vi "Create All Message Queues.vi"(8 "error in (no error)":errorcluster) -> (0 "error out":errorcluster, 3 "Message Queues out":T1)   [LabVIEW 2018, in "Message Queue.lvlib"]
doc: "This VI creates and initializes all the message queues for your application. If your application requires more than one message queue, right-click the \"Message Queues\" constant above and select Open Type Def. Add the new Message Queue(s) to the type definition, then initialize them in this VI."
uses:
  Message Queue.lvlib
  All Message Queues.ctl
  Message Cluster (enum).ctl
  Message (enum).ctl
  Message Cluster (string).ctl
  Enqueue Message (string).vi
  Enqueue Message (enum).vi
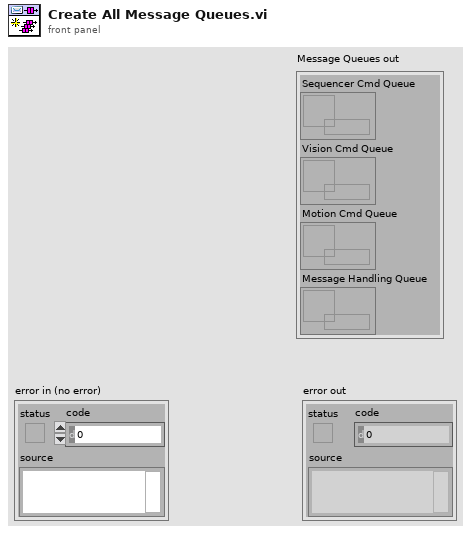
[diagram p1: front panel]
types:
  T1 = typedef "Message Queue.lvlib/All Message Queues.ctl" = cluster{"Sequencer Cmd Queue":refnum<queue>, "Vision Cmd Queue":refnum<queue>, "Motion Cmd Queue":refnum<queue>, "Message Handling Queue":refnum<queue>}
  T2 = typedef "Message Queue.lvlib/Message (enum).ctl" = enum16{"Initialize", "Idle", "Running", "Stop", "Pause", "Resume", "Load Sequence", "Exit"}
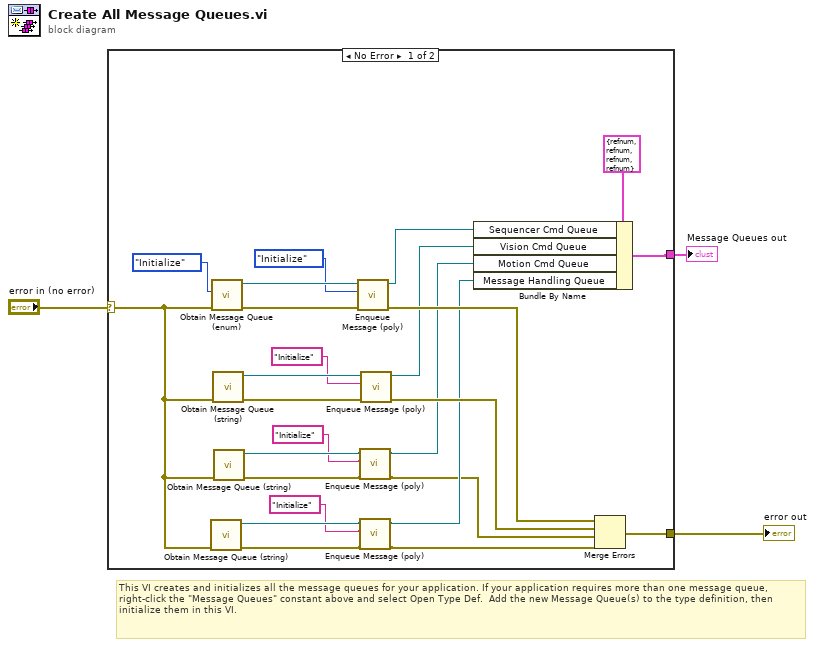
[diagram p0: block diagram]
diagram:
  # "This VI creates and initializes all the message queues for your application. If your application requires more than one message queue, right-click the \"Message Queues\" constant above and select Open Type Def.  Add the new Message Queue(s) to the type definition, then initialize them in this VI."
  n1 = case shown="No Error" "error in (no error)" {
    selector: "error in (no error)" -> [w5 w29]
    tunnel: [w26 w29] -> w3
    tunnel: [w27 _] -> w2
    frame No Error {
      n2 = call "Obtain Message Queue (string).vi"("error in (no error)"=w5) -> ("error out"=w13:errorcluster, "queue out"=w14:refnum<queue>)  [unwired: 9 in]
      n3 = call "Obtain Message Queue (enum).vi"("error in (no error)"=w5, "Message"=Message_(enum)."Initialize" ("Enum")) -> ("error out"=w25:errorcluster, "queue out"=w23:refnum<queue>)  [unwired: 8 in]
      n4 = call "Obtain Message Queue (string).vi"("error in (no error)"=w5) -> ("error out"=w20:errorcluster, "queue out"=w19:refnum<queue>)  [unwired: 9 in]
      n5 = call "Obtain Message Queue (string).vi"("error in (no error)"=w5) -> ("error out"=w9:errorcluster, "queue out"=w17:refnum<queue>)  [unwired: 9 in]
      n6 = call-poly "Enqueue Message (poly).vi"("error in (no error)"=w25, "Enum"=Message_(enum)."Initialize", "Message Queue"=w23) -> ("error out"=w24:errorcluster, "dup Message Queue"=w6:refnum<queue>)  [unwired: 7 in]
      n7 = call-poly "Enqueue Message (poly).vi"("error in (no error)"=w9, "Message"="Initialize", "Message Queue"=w17) -> ("error out"=w8:errorcluster, "dup Message Queue"=w16:refnum<queue>)  [unwired: 7 in]
      n8 = call-poly "Enqueue Message (poly).vi"("error in (no error)"=w13, "Message"="Initialize", "Message Queue"=w14) -> ("error out"=w12:errorcluster, "dup Message Queue"=w15:refnum<queue>)  [unwired: 7 in]
      n9 = call-poly "Enqueue Message (poly).vi"("error in (no error)"=w20, "Message"="Initialize", "Message Queue"=w19) -> ("error out"=w21:errorcluster, "dup Message Queue"=w22:refnum<queue>)  [unwired: 7 in]
      n10 = Bundle By Name(cluster=T1 {"Sequencer Cmd Queue"=refnum, "Vision Cmd Queue"=refnum, "Motion Cmd Queue"=refnum, "Message Handling Queue"=refnum} ("Message Queues"), "Sequencer Cmd Queue"=w6, "Vision Cmd Queue"=w22, "Motion Cmd Queue"=w16, "Message Handling Queue"=w15) -> (w27:T1)
      n11 = Merge Errors(w24, w21, w8, w12) -> (w26:errorcluster)
    }
    frame Error {
    }
  }
  "Message Queues out" <- w2
  "error out" <- w3
